vi "acces.vi"() -> ()   [LabVIEW 2015]
uses:
  <vilib>/httpClient/LabVIEWHTTPClient.lvlib
panel:
  in  "Boolean 6":bool
  in  "Boolean 5":bool
  in  "Boolean 4":bool
  in  "Boolean 3":bool
  in  "Boolean 2":bool
  in  "Boolean":bool
  in  "Boolean":bool
  in  "OK Button 4":bool
  in  "Combo Box":string(combo)
  in  "OK Button":bool
  # "Choisir  Cin utilisateur"
  # "Commande"
  # "Supervision"
  # "Scenarios"
  # "Gestion Chambre"
  # "Gestion Utilisateur"
  # "Gestion Equipement"
  # "Droits Accès"
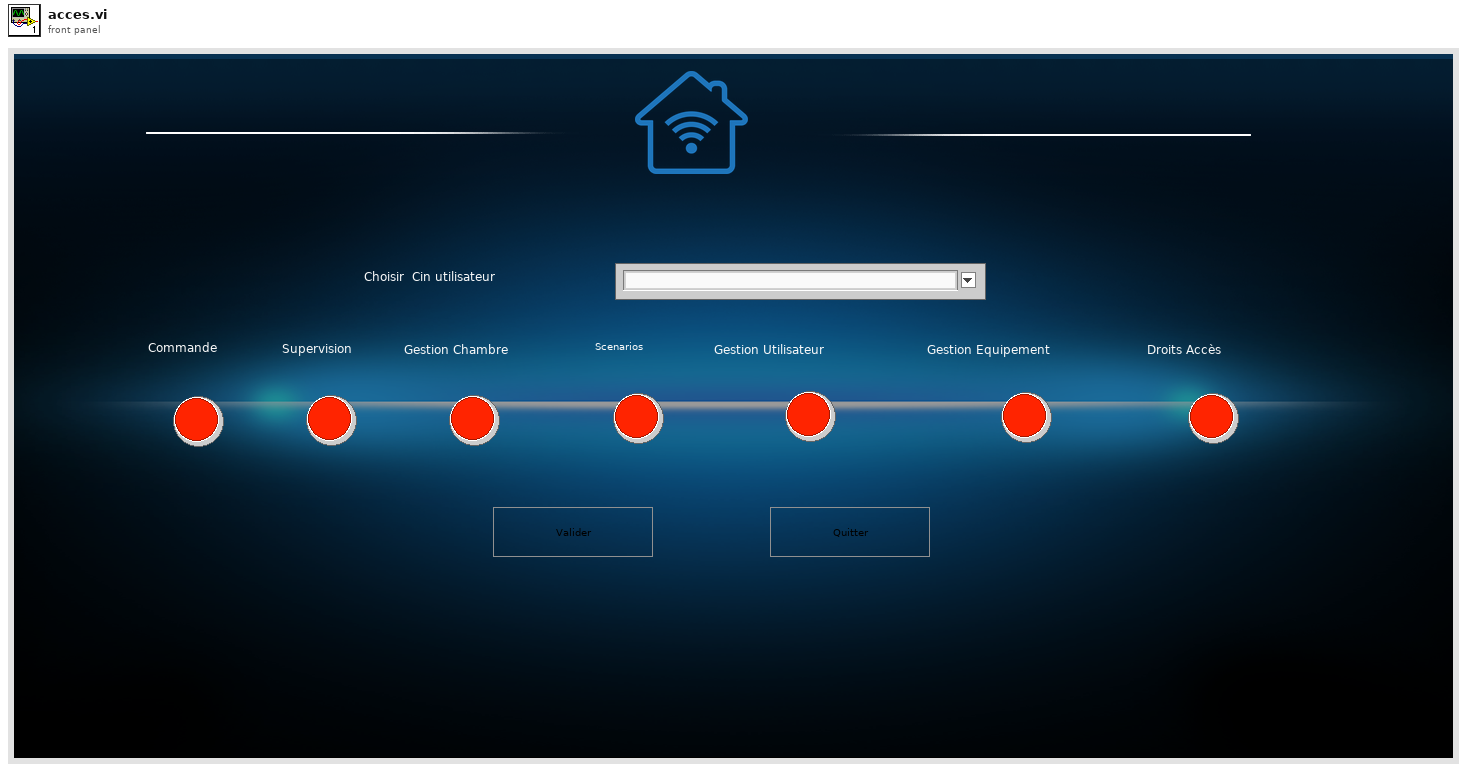
[diagram p1: front panel]
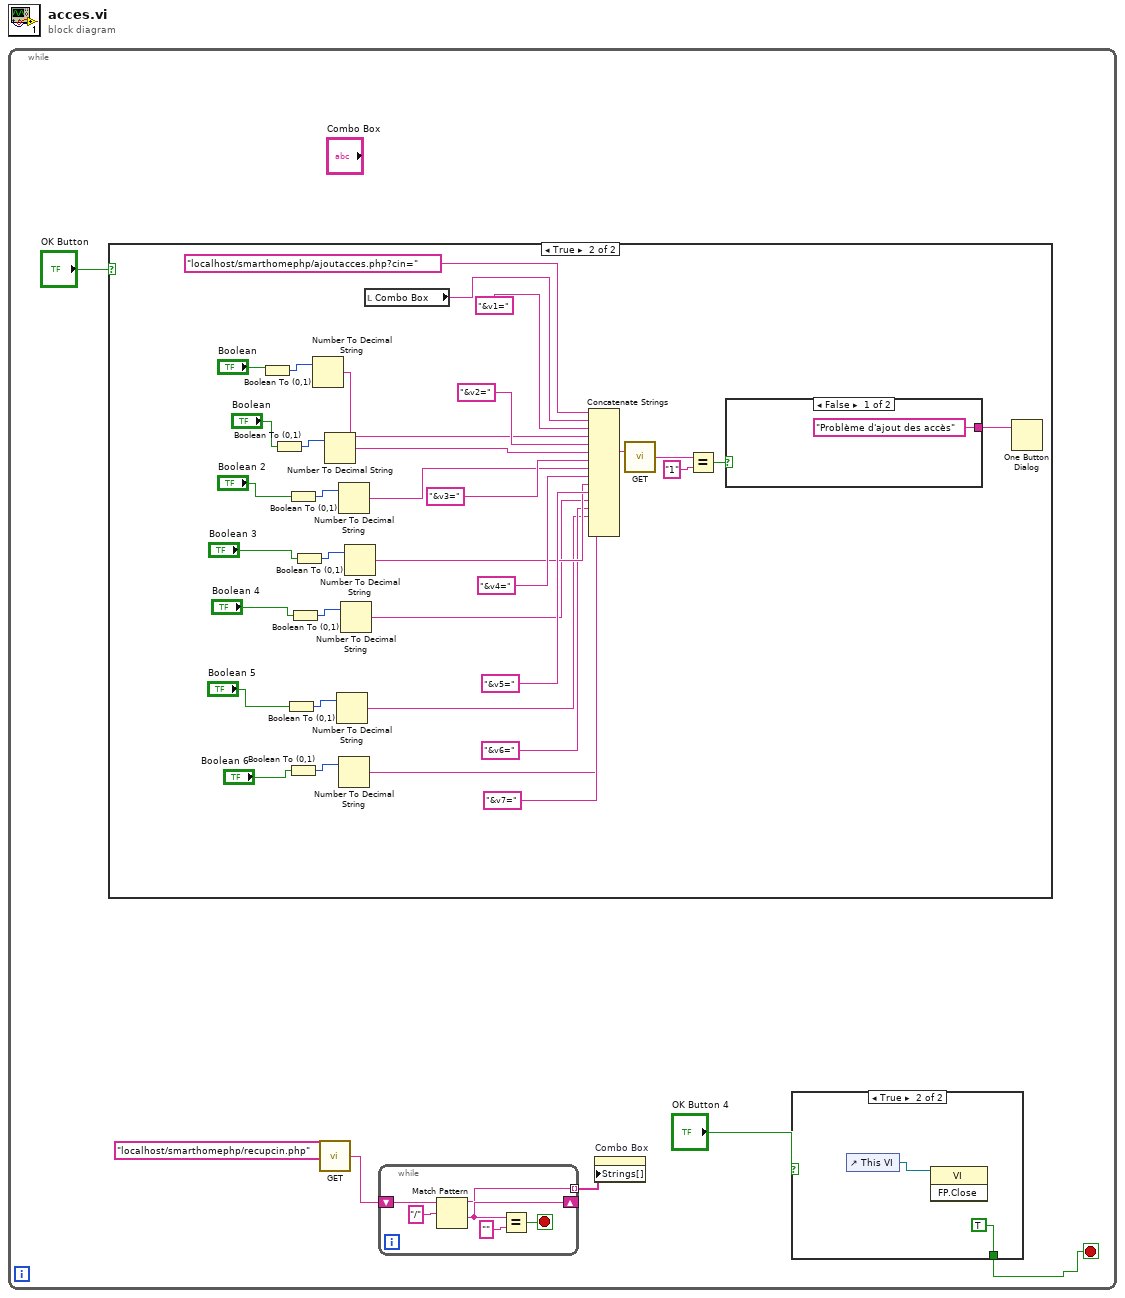
[diagram p0: block diagram]
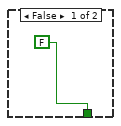
[diagram p2: hidden frame]
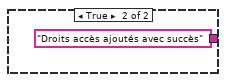
[diagram p4: hidden frame]
diagram:
  n1 = while {
    stop <- w1 stop-if-true
    n2 = case shown="True" "OK Button" {
      frame False {
      }
      frame True {
        n3 = Boolean To (0,1)(Boolean="Boolean") -> (0, 1=w37:i16)
        n4 = Boolean To (0,1)(Boolean="Boolean") -> (0, 1=w35:i16)
        n5 = Boolean To (0,1)(Boolean="Boolean 5") -> (0, 1=w31:i16)
        n6 = Boolean To (0,1)(Boolean="Boolean 2") -> (0, 1=w34:i16)
        n7 = Boolean To (0,1)(Boolean="Boolean 6") -> (0, 1=w30:i16)
        n8 = Boolean To (0,1)(Boolean="Boolean 4") -> (0, 1=w32:i16)
        n9 = Boolean To (0,1)(Boolean="Boolean 3") -> (0, 1=w33:i16)
        n10 = Number To Decimal String(number=w37) -> (decimal integer string=w36:string)  [unwired: 1 in]
        n11 = Number To Decimal String(number=w35) -> (decimal integer string=w29:string)  [unwired: 1 in]
        n12 = Number To Decimal String(number=w31) -> (decimal integer string=w24:string)  [unwired: 1 in]
        n13 = Number To Decimal String(number=w34) -> (decimal integer string=w28:string)  [unwired: 1 in]
        n14 = Number To Decimal String(number=w30) -> (decimal integer string=w22:string)  [unwired: 1 in]
        n15 = Number To Decimal String(number=w32) -> (decimal integer string=w26:string)  [unwired: 1 in]
        n16 = Number To Decimal String(number=w33) -> (decimal integer string=w27:string)  [unwired: 1 in]
        n17 = local read "Combo Box"() -> (w49:string)
        n18 = Concatenate Strings("localhost/smarthomephp/ajoutacces.php?cin=", w49, "&v1=", w36, "&v2=", w29, "&v3=", w28, "&v4=", w27, "&v5=", w26, "&v6=", w24, "&v7=", w22) -> (w43:string)
        n19 = call <vilib>:"GET.vi"("url"=w43) -> ("body"=w42:string)  [unwired: 11 in, 3 out]
        n20 = Equal?(x=w42, y="1") -> (x = y?=w40:bool)
        n21 = case shown="False" w40 {
          tunnel: ["Problème d'ajout des accès" "Droits accès ajoutés avec succès"] -> w39
          frame False {
          }
          frame True {
          }
        }
        n22 = One Button Dialog(message=w39) -> ()  [unwired: 1 in, 1 out]
      }
    }
    n23 = call <vilib>:"GET.vi"("url"="localhost/smarthomephp/recupcin.php") -> ("body"=w4:string)  [unwired: 11 in, 3 out]
    n24 = while {
      shift-right: [w12] -> _
      shift-left: w4 -> [w14]
      tunnel: [w10] -> w5 mode=indexing
      stop <- w11 stop-if-true
      n25 = Match Pattern(string=w14, regular expression="/") -> (before substring=w10:string, after substring=w12:string)  [unwired: 1 in, 2 out]
      n26 = Equal?(x=w12, y="") -> (x = y?=w11:bool)
    }
    n27 = property on="Combo Box" class="CmbBox"("Strings[]"=w5) -> ()  [unwired: 2 in, 2 out]
    n28 = case shown="True" "OK Button 4" {
      tunnel: [FALSE TRUE] -> w1
      frame False {
      }
      frame True {
        n29 = control-ref of="This VI"() -> (w9:refnum<vi>)
        n30 = invoke class="VI" method="FP.Close"(reference=w9) -> ()  [unwired: 2 in, 3 out]
      }
    }
  }
